vi "_Number Count Down(Element).vi"(0 "number":i32, 1 "reset(F)":bool, 2 "threashold":i64=1000, 3 "Valid?(T)":bool) -> (6 "reach?":bool, 9 "left":i64)   [LabVIEW 2017]
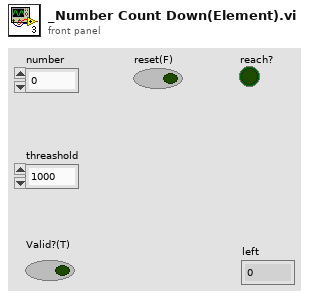
[diagram p1: front panel]
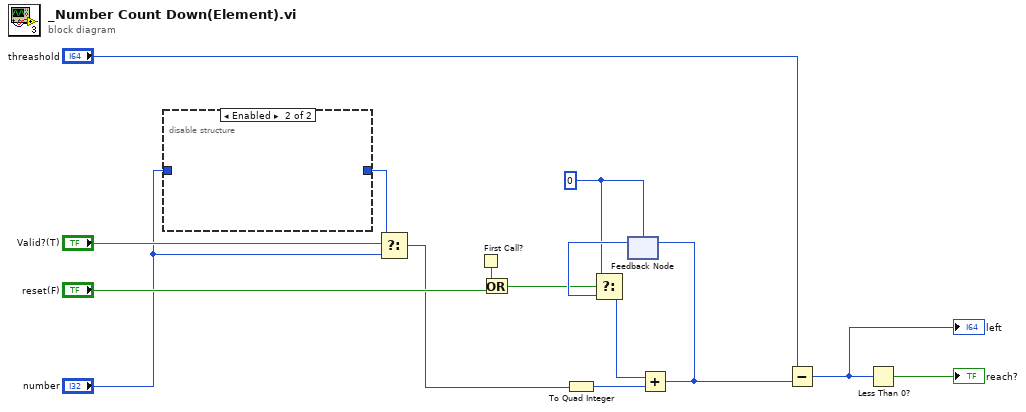
[diagram p0: block diagram]
diagram:
  w6 = i64 0 ("t")
  n1 = disable-structure shown="Enabled" {
    disable-tunnel: "number" -> [w16 _]
    disable-tunnel: [w16 _] -> w1
    frame Disabled {
    }
    frame Enabled {
    }
  }
  n2 = Select(t=w1, s="Valid?(T)", f="number") -> (s? t:f=w3:i32)
  n3 = First Call?() -> (First Call?: T/F=w11:bool)
  n4 = Or(x=w11, y="reset(F)") -> (x .or. y?=w10:bool)
  n5 = To Quad Integer(1:w3) -> (0:w5:i64)
  n6 = feedback #1(w6) -> (w15:i64)
  n7 = Select(t=w6, s=w10, f=w15) -> (s? t:f=w12:i64)
  n8 = Add(x=w12, y=w5) -> (x+y=w13:i64)
  n9 = feedback-in #1(w13) -> ()
  n10 = Subtract(x="threashold", y=w13) -> (x-y=w8:i64)
  "left" <- w8
  n11 = Less Than 0?(x=w8) -> (x < 0?=→"reach?":bool)
